vi "Splash Screen.vi"(8 "error in":errorcluster) -> (0 "error out":errorcluster)   [LabVIEW 2020, in "Panther Dashboard.lvlib"]
uses:
  Panther Dashboard.lvlib
panel:
  out "Pdash Version":string
  out "Progress":u16(slide) scale=-1.0..30.0
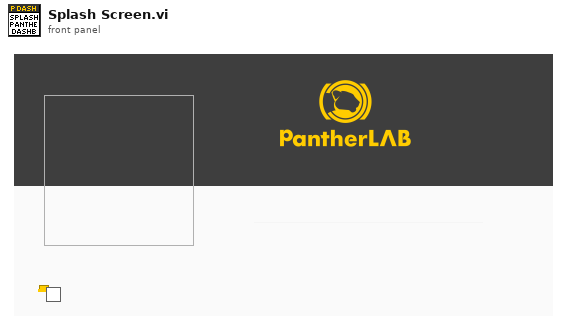
[diagram p1: front panel]
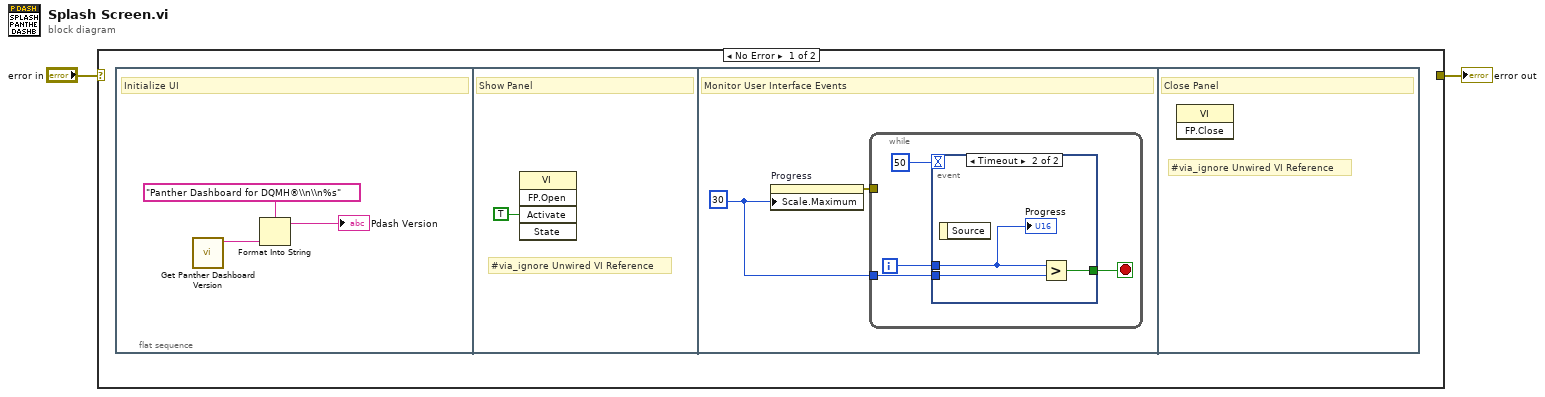
[diagram p0: block diagram]
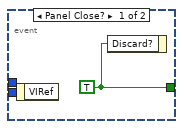
[diagram p2: hidden frame]
diagram:
  n1 = case shown="No Error" "error in" {
    selector: "error in" -> [_ w17]
    tunnel: [_ w17] -> w1
    frame No Error {
      n2 = flat-sequence {
        frame #0 {
          # "Initialize UI"
          n3 = call "Get Panther Dashboard Version.vi"() -> ("Panther Dashboard Version"=w3:string)  [unwired: 11 in]
          n4 = Format Into String(format string="Panther Dashboard for DQMH®\\n\\n%s", w3) -> (resulting string=→"Pdash Version":string)  [unwired: 2 in, 1 out]
        }
        frame #1 {
          # "#via_ignore Unwired VI Reference"
          # "Show Panel"
          n5 = invoke class="VI" method="FP.Open"("Activate"=TRUE ("Activate?")) -> ()  [unwired: 4 in, 5 out]
        }
        frame #2 {
          w7 = 30 ("y")
          # "Monitor User Interface Events"
          n6 = property on="Progress" class="Slide (strict)"("Scale.Maximum"=w7) -> (error out=w8:errorcluster)  [unwired: 2 in, 1 out]
          n7 = while {
            tunnel: w8 -> [_]
            tunnel: w7 -> [w9]
            i -> [w11]
            stop <- w12 stop-if-true
            n8 = event shown="[1] Timeout" {
              selector: _ -> [_ _]
              dyn-events: _ -> [_ _]
              timeout: 50 -> [_ _]
              tunnel: [w13 w16] -> w12
              tunnel: w11 -> [_ w15]
              tunnel: w9 -> [_ w14]
              event Panel Close? {
                w13 = TRUE ("Discard?")
                n9 = event-data() -> ()  [unwired: 1 in, 1 out]
                n10 = event-data("Discard?"=w13) -> ()  [unwired: 1 in, 1 out]
              }
              event Timeout {
                n11 = event-data() -> ()  [unwired: 1 in, 1 out]
                n12 = Greater?(x=w15, y=w14) -> (0:w16:bool)
                "Progress" <- w15
              }
            }
          }
        }
        frame #3 {
          # "#via_ignore Unwired VI Reference"
          # "Close Panel"
          n13 = invoke class="VI" method="FP.Close"() -> ()  [unwired: 3 in, 3 out]
        }
      }
    }
    frame Error {
    }
  }
  "error out" <- w1
